vi "Day 2 task 1.vi"() -> ()   [LabVIEW 2022 SP3]
uses:
  <vilib>/regexp/Match Regular Expression.xnode
panel:
  out "sum":i32
  out "Array":i32[](array[numeric])
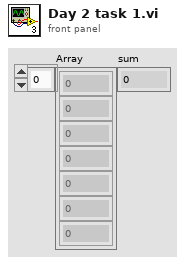
[diagram p1: front panel]
types:
  T1 = cluster{"Mine":string, "Theirs":string, "Score":i32}[]
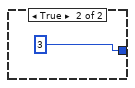
[diagram p2: hidden frame]
diagram:
  (unwired) "A Y\nB X\nC Z"
  w9 = TRUE ("replace all? (F)")
  n1 = Search and Replace String(replace all?=w9, input string="C Y\nC Y\nB Y\nA Z\nB Z\nA X\nA Y\nA Y\nA X\nA Y\nB Y\nA Y\nB Y\nB Y\nB Z\nB Z\nB Z\nB Z\nA Y\nB Z\nA Y\nB X\nB Y\nB X\nA X\nA X\nB Z\nA X\nA X\nB Z\nB Z\nB Y\nB Z\nB Z\nB Z\nB Y\nA X\nA X\nB Z\nA X\nB X\nB X\nC Y\nB Z\nC X\nA X\nA Y\nB Y\nA Y\nB X\nA X\nB Y\nB Z\nB Z\nB Y\nB Z\nC Z\nB X\nB X\nB Z\nB Z\nB Z\nB Z\nA Y\nB X\nA X\nC X\nB Y\nB Z\nA Y\nB Z\nB Z\nB Y\nB Y\nB Z\nB Y\nB Z\nA X\nB X\nB X\nA X\nA X\nB Z\nB Z\nB Z\nB Z\nB Y\nB X\nB Z\nA X\nA Y\nB Z\nA Y\nB Z\nB Y\nB Z\nA X\nB Y\nA Y\nB Z\nA Z\nA Y\nA Y\nC Y\nB Z\nB X\nA Z\nB Z\nA X\nB Z\nA Z\nB Z\nA X\nB Y\nA X\nB Y\nB Z\nB X\nB X\nB Z\nB Z\nB Z\nA X\nB Z\nA X\nB X\nB Z\nA X\nC Z\nB Z\nB Z\nB Y\nB Y\nB Y\nB Z\nB Z\nA Y\nB Z\nB Z\nC Y\nC Z\nA X\nB Z\nB X\nB Z\nB Z\nB Y\nA X\nB Z\nB Y\nA Z\nB Z\nA X\nA X\nB Y\nA Y\nB Z\nB Z\nB X\nB Y\nA X\nA Y\nB X\nC Z\nA Y\nB Z\nB Z\nB Z\nA Z\nC Y\nB Y\nB Y\nB Z\nC Y\nB Y\nB X\nB X\nB Z\nC Z\nA X\nB Z\nB Z\nB Z\nB Z\nB X\nB X\nA X\nA Z\nA Z\nA X\nC Y\nB X\nA X\nA Y\nA X\nB X\nA Y\nB Z\nB Z\nA Y\nA X\nB Y\nB Z\nB Z\nA X\nA Z\nB Z\nB X\nA X\nB Z\nB Y\nA Y\nA Z\nB X\nA Y\nB Z\nA Z\nB Z\nA Y\nB Z\nB X\nB Y\nA Y\nB Z\nB Z\nA X\nA X\nB Y\nB Z\nA X\nB Z\nB Z\nB Z\nB Z\nB Z\nA Z\nB Z\nB Z\nB X\nA Y\nC X\nB Z\nB Y\nB Y\nB Z\nB Z\nB Z\nB Y\nB X\nB Y\nC X\nB Z\nA Z\nA Y\nC X\nA X\nB X\nA X\nB X\nA Y\nB Z\nA Y\nA Y\nB Z\nB X\nB Z\nA Y\nB Z\nB X\nC Z\nC X\nC Z\nB Y\nB X\nB Z\nB Z\nB Y\nB Z\nB Y\nB Z\nA X\nB X\nB Z\nA X\nB Z\nB Y\nB Z\nA X\nB Y\nC Y\nA Z\nB Z\nC Z\nA Y\nB Z\nA Y\nA Z\nB Y\nA X\nA X\nB Z\nB Z\nB Z\nA Y\nB Z\nA Z\nB Z\nA Y\nA Z\nB Y\nC Z\nB Z\nA Z\nB X\nB Z\nB Y\nB Z\nA Z\nA Z\nB Z\nB X\nC Z\nB X\nB Z\nB Y\nA X\nB Z\nA X\nB X\nB Z\nB Z\nA X\nB X\nC X\nC X\nB X\nB Y\nB Z\nB X\nB Y\nB Y\nB Z\nA Z\nB Z\nC X\nA Y\nC X\nB Z\nA Y\nB Z\nB Y\nB Z\nB X\nA X\nB X\nB Z\nA Y\nA Y\nB Z\nB Z\nB Z\nA Y\nB Z\nB X\nC X\nB Z\nB Z\nC Y\nB Z\nC Y\nB Z\nC Y\nC X\nB Z\nC Y\nA Y\nA Y\nC Z\nB Z\nB X\nB Z\nB X\nC Z\nB Z\nA Z\nB Z\nC Y\nB Z\nA X\nA Y\nB Y\nB Y\nB Z\nA Y\nB X\nB Z\nB Z\nA Z\nB X\nA Y\nA Y\nB Z\nB Z\nB Z\nC X\nA Z\nB X\nC Z\nB Y\nB Z\nB X\nA Y\nB Z\nA X\nB X\nB Y\nA Y\nB Z\nB Z\nB Y\nA Z\nB Z\nA X\nB Y\nA Y\nA X\nA Y\nA X\nA X\nB X\nB Y\nB X\nB Y\nB Z\nB Y\nB X\nA X\nB Z\nA Z\nA X\nB Z\nB Y\nA X\nB Y\nA X\nB X\nC Y\nB X\nB X\nB X\nC Y\nB X\nB Y\nB Y\nB Y\nB Y\nB X\nA Y\nC Y\nB Z\nB Z\nB X\nB Z\nC Y\nB Y\nB Z\nB Z\nB Y\nB Z\nA X\nB X\nB Y\nA X\nC Y\nB Z\nA Y\nB Z\nB Z\nB Z\nA X\nB Y\nB Z\nB Y\nB Z\nA X\nB Z\nA X\nB Y\nB Y\nB X\nB X\nA Y\nB Z\nC Y\nA X\nA X\nB X\nB Z\nB X\nB X\nB Z\nB Z\nA X\nB X\nB Z\nA Z\nB Y\nA X\nB Z\nC Y\nB Z\nB X\nB Z\nB Z\nA Y\nA Y\nB Z\nB X\nB Y\nB Z\nA Y\nA Y\nB X\nB X\nC X\nB Z\nC Z\nB X\nA Y\nB Z\nA Z\nB Y\nA Y\nB Z\nB X\nB X\nA Y\nB Z\nB Y\nA X\nB Y\nB Y\nB Y\nB X\nB Y\nB Z\nB Y\nB Y\nA X\nC Z\nB Z\nB Z\nA Z\nB Z\nB Z\nA X\nB X\nA Y\nA X\nB X\nC X\nB X\nB Z\nB Y\nA Z\nA Y\nB Y\nB Z\nB X\nB X\nB Z\nB Z\nB Y\nA X\nB Z\nA Y\nA X\nB Y\nB Z\nB Z\nB X\nA X\nA Y\nC X\nA Y\nB Z\nB Y\nB Z\nB Z\nC Z\nB Z\nB X\nA X\nC Y\nB X\nB Z\nA Z\nA X\nA Y\nB Z\nB Z\nA Y\nA Y\nB X\nA Y\nA Y\nB Z\nA Y\nB Y\nB Z\nA Y\nA Z\nB X\nB X\nB Y\nB Z\nB Z\nA X\nB X\nC X\nB Y\nA Y\nA X\nA X\nA X\nB Y\nA X\nA Z\nA Y\nB X\nA Y\nB Z\nC X\nB X\nB X\nB Z\nB X\nB X\nB Z\nA X\nB Z\nB X\nB Z\nA Y\nB Y\nB Z\nB Y\nB Z\nB Z\nA X\nB Z\nA Y\nC Z\nA Y\nB Z\nA Y\nB X\nB Z\nB X\nC Y\nA X\nB Z\nB Y\nA X\nA X\nB X\nB Z\nA Z\nB Z\nB X\nB X\nB X\nB Z\nB Z\nB Y\nB X\nB X\nA X\nB Z\nB X\nA X\nA X\nA X\nB X\nB Z\nA Z\nB X\nB Y\nB Y\nB Z\nB Z\nC Z\nA Y\nA X\nB Y\nB X\nB Z\nB X\nA X\nB Z\nB Z\nB Y\nB Z\nB X\nB Z\nB Z\nB X\nB X\nA X\nA X\nB X\nB Z\nB Z\nC X\nC X\nB Z\nB Z\nB X\nB Z\nB Y\nB X\nA X\nB Y\nA Y\nA X\nB Z\nB Z\nC X\nB Y\nB Z\nB Z\nB X\nB Z\nB Z\nC Z\nB Z\nB Y\nB Z\nB X\nA X\nB X\nB Z\nB Z\nA Y\nB Z\nB Z\nB Z\nB Z\nA X\nB Z\nB Z\nB X\nB Y\nB Y\nB Z\nA X\nB Z\nB Y\nB X\nA X\nB X\nB Z\nB Z\nB Z\nB X\nB Z\nB Z\nB Z\nA Y\nB Z\nC X\nB Y\nB Y\nB Y\nA Y\nB Z\nB Z\nA X\nC Z\nB Z\nB Z\nB Z\nB X\nB Z\nA Z\nB Z\nB Z\nB Z\nA Z\nB Z\nC Y\nB X\nA X\nA Y\nB Z\nB Z\nA Z\nB Z\nB X\nA Z\nB Y\nB Z\nB X\nB Z\nB X\nB Y\nB Z\nA X\nB Z\nB Z\nA Y\nB X\nB X\nB X\nA Z\nC X\nA Z\nB Z\nB Z\nB Z\nB X\nA Y\nC X\nA Z\nA Y\nB X\nB Z\nB X\nB Z\nB Y\nA Y\nB X\nC X\nA Y\nC Z\nA X\nB Z\nB Z\nA Z\nB X\nB Y\nB Z\nA Y\nB Y\nA X\nA X\nC Y\nA Y\nB X\nA X\nB Y\nB X\nB Y\nA Y\nA X\nC Y\nB Y\nB Y\nB Z\nB Y\nB X\nB Z\nB Z\nB X\nA X\nB Z\nB Z\nB Z\nB X\nB Z\nB X\nB Z\nB Z\nB Y\nB Y\nB X\nA X\nB Z\nB Y\nA Y\nB Z\nB X\nB Z\nB Z\nA Z\nB Z\nA Y\nB Z\nA X\nB Z\nB Z\nA Y\nB Z\nA X\nB Z\nA Y\nA Y\nA Z\nB X\nB Z\nB Y\nA Z\nC Z\nB Z\nA X\nA X\nB X\nA Z\nB X\nB X\nB Z\nC X\nB Z\nB Z\nB Z\nB Z\nB X\nA Z\nA Y\nB Z\nB Y\nC Z\nB Y\nB Z\nA Y\nB X\nB X\nB Z\nA X\nA Y\nB Z\nB X\nB Y\nA Y\nC Y\nC Y\nB Z\nA Y\nB Y\nA Y\nB Z\nB Z\nA X\nB X\nA X\nB X\nA Y\nA X\nB Z\nA X\nB Z\nB X\nB Z\nB X\nB X\nA X\nA Y\nB Z\nB X\nB X\nA X\nA Y\nA X\nB Y\nB Z\nB Z\nB Z\nB Z\nB Z\nB X\nB Y\nA Y\nB X\nB Z\nA Y\nB X\nA X\nB Z\nC X\nB Y\nA Y\nA X\nA X\nB X\nB X\nB Z\nB Z\nB Z\nB X\nB Y\nB X\nB Z\nB X\nB Y\nB X\nB Z\nB X\nB Y\nB X\nB Z\nB Z\nB Z\nA X\nC X\nC Y\nA Y\nB X\nB X\nA Y\nB Z\nB X\nB Z\nB X\nB X\nC X\nB Z\nB Z\nB Y\nA Z\nA Z\nC X\nB X\nC Y\nB Z\nC X\nB Z\nA Y\nC Z\nB X\nB Y\nA Y\nB Y\nB X\nB Z\nA Y\nA Z\nC X\nB Z\nA X\nB X\nB Z\nC Z\nA Y\nB Z\nB Z\nA X\nA X\nB Z\nB Y\nC Z\nB Z\nB X\nB Z\nA X\nA X\nB Y\nA X\nB X\nA Y\nB Z\nA Y\nB Z\nA Y\nB Z\nA X\nB Y\nB Z\nB Z\nB Z\nA X\nA X\nB X\nB Z\nA X\nB Z\nA X\nA X\nB Z\nB Z\nB Z\nB X\nB Y\nB Z\nB Z\nB X\nB Z\nB Y\nB Z\nC Y\nB X\nC Z\nB Z\nB Z\nA Y\nB Z\nB X\nA Y\nB Z\nB X\nB Z\nB Z\nB Y\nB Z\nA Z\nA Y\nB Z\nB Z\nB Y\nA Y\nB Z\nA X\nB X\nA Z\nA X\nB X\nB Z\nB X\nB Z\nB Z\nB Y\nB Y\nB Z\nB Y\nB Z\nB Z\nA X\nB X\nB Y\nB Y\nC Z\nA X\nB Y\nA Y\nB Z\nB Z\nB Z\nC X\nB X\nA Z\nB Y\nA X\nC X\nB Z\nB Z\nB Z\nB Y\nA Y\nA Y\nB Y\nB Z\nB Z\nB Z\nC X\nA X\nB Z\nA Y\nB X\nB Z\nB Z\nB Z\nB Z\nB X\nB Y\nB Z\nB Z\nA Y\nC X\nA X\nB Z\nB Z\nA Y\nA Y\nB Z\nA Y\nB Y\nA X\nB Z\nB Z\nA Y\nB Z\nB Z\nA X\nA X\nB X\nB Z\nB Z\nA X\nB Z\nB Z\nC Y\nB Z\nA X\nB Z\nA X\nB Z\nA X\nB X\nA X\nA Y\nB Z\nB X\nA X\nB Z\nA X\nA Z\nB Z\nB Z\nB Z\nA Y\nB X\nA X\nB Y\nA Y\nB Z\nB Z\nB X\nB Z\nB X\nB X\nA X\nB Z\nA Y\nA X\nB X\nA Z\nB X\nB Y\nB Z\nB X\nB X\nB Z\nC X\nA X\nB Z\nB Y\nC Z\nB Z\nA Z\nA Z\nA X\nA Y\nB Z\nB Z\nB X\nA Z\nB Z\nB Z\nB X\nB Y\nB X\nB Z\nB X\nB Z\nA Y\nA X\nB Z\nB X\nB Y\nB Z\nB Z\nB Z\nB Z\nC X\nC X\nB Z\nB X\nB Z\nB Z\nB Z\nB X\nB Z\nB Z\nB Z\nB X\nB Z\nB Z\nB Z\nC Y\nB Z\nB Y\nB Z\nA Z\nA Y\nB Z\nA Y\nC X\nA X\nB X\nA Y\nB Z\nA Y\nB Z\nB Y\nB Z\nB Z\nC Y\nB Y\nB Z\nB Z\nB X\nB Y\nB Z\nB Y\nB Z\nB X\nB Y\nB Z\nB Z\nB Z\nB Y\nB Y\nB Z\nB Z\nC X\nB Z\nA Y\nB Z\nB Z\nB Y\nB Y\nB Z\nB Z\nA Y\nB Z\nA Z\nC X\nA Y\nA Y\nA X\nB Z\nA X\nC Y\nA Z\nC Y\nC X\nB Z\nA X\nA Y\nB Z\nB Z\nB Z\nB Z\nB Y\nA Z\nA Y\nB Y\nA Y\nA Z\nB X\nB Z\nB Z\nA X\nC Y\nB Z\nB X\nC X\nA Z\nB Z\nB X\nB Y\nA X\nA X\nB Z\nC X\nB Z\nB Z\nB X\nB Z\nB Z\nB Z\nA X\nB Z\nB Y\nB Z\nB Z\nB Y\nB X\nA X\nB Z\nA X\nA X\nB Y\nB Z\nB X\nA Y\nC X\nB Y\nA X\nA X\nA X\nC Y\nB X\nC Z\nA X\nB Z\nA Z\nB Z\nA X\nA Y\nB Z\nA X\nB X\nA Y\nA X\nA Y\nB X\nB Y\nB Z\nB Y\nC X\nC Y\nB Z\nB Y\nB Z\nA X\nC Z\nB Z\nA X\nB X\nA X\nB X\nB Z\nB X\nB Z\nB Z\nB Z\nA X\nA X\nB Z\nB X\nB Z\nB Z\nB Z\nA X\nB Z\nB X\nA X\nC Z\nA Y\nB Z\nA Y\nB Z\nB Z\nB Z\nC Z\nB Z\nB Z\nA X\nB X\nA X\nB X\nA X\nB Z\nB Z\nB X\nB Z\nA X\nA Y\nA Y\nA Y\nB Z\nB Z\nB Z\nB Z\nA X\nB Z\nB Z\nB Y\nB Z\nA Z\nB Z\nA Y\nB Y\nB Y\nC Y\nB X\nB Z\nB Y\nB Z\nB Y\nB Z\nB Z\nA Y\nB X\nA Z\nB Z\nA X\nB Y\nA X\nB Z\nB Y\nA X\nB X\nB Z\nB Z\nB Z\nA Y\nA Y\nA X\nA Y\nA Y\nB X\nB Z\nB Y\nB Y\nB X\nB Y\nB X\nB X\nB X\nB Z\nB Z\nB Z\nA Y\nA Z\nB Y\nC X\nB X\nB Z\nC Y\nB Z\nC Y\nB Z\nB Z\nB Z\nB X\nA X\nB Z\nB Z\nA X\nB Z\nB Z\nB Z\nB Z\nB Z\nB Z\nB X\nA X\nA Y\nB Y\nB Z\nB Y\nB X\nA Z\nA X\nB X\nB Y\nB Z\nB Z\nB Z\nB X\nC X\nB X\nA Z\nA X\nA Y\nB Z\nB Z\nA X\nB Z\nA Y\nB X\nB Z\nB Y\nB Y\nA X\nB X\nB Z\nB Z\nB Z\nB Z\nB Y\nA Z\nA Y\nB X\nA X\nB Y\nB Z\nC Y\nB Z\nB Z\nB X\nA Z\nA Y\nB Y\nB Z\nA Y\nB Y\nA Y\nA X\nA Y\nB Y\nC X\nC Z\nB X\nA Z\nA X\nB Y\nB X\nA X\nB Z\nA Y\nA Z\nB Z\nB Z\nB Z\nA X\nB Z\nB Y\nB Z\nA X\nA Y\nB Z\nB X\nC X\nB Z\nA Y\nB Z\nB Z\nB X\nB Z\nB Z\nA Y\nA X\nB Z\nC Y\nA Y\nB Y\nB Z\nA X\nB Z\nB Z\nB Z\nB Z\nC X\nB Y\nB Z\nB X\nB Z\nB Z\nB Z\nB Z\nB Z\nB Y\nA X\nB Y\nA Y\nA X\nA X\nB Z\nB Z\nB Z\nC X\nB X\nB Z\nA X\nA X\nB Y\nA X\nB Z\nB Z\nB X\nB Y\nB Y\nB Y\nA Y\nA Y\nA X\nA X\nB Z\nB Y\nB Y\nB X\nB Y\nB Z\nA Z\nB Z\nA Z\nB X\nB Y\nC Y\nB X\nB X\nA X\nA X\nA X\nA X\nB Z\nB Z\nA Z\nB X\nB X\nB X\nB X\nB X\nB Z\nB Z\nB Z\nB Z\nB Z\nB Y\nB Z\nB Z\nA Y\nA Z\nC Y\nB Y\nA X\nB Z\nB X\nA Y\nB Y\nA Y\nC Z\nA X\nA Y\nB X\nB X\nC Z\nB Y\nA Y\nA Y\nA X\nB X\nA X\nB X\nA Y\nB Z\nB Z\nA Z\nB X\nB Z\nB Z\nB Y\nA Y\nB Z\nB Y\nB Z\nB Z\nB Z\nC X\nB Y\nA Y\nB Z\nA Y\nA Y\nA X\nB X\nB Y\nC Y\nC X\nB Z\nB Z\nB Z\nA Y\nA Z\nB Y\nB X\nB X\nB Y\nB Z\nB Z\nA Y\nB Y\nB Z\nB Z\nB Z\nA X\nC Y\nB Z\nA Z\nC Z\nB X\nB Y\nB Z\nA Z\nA X\nB X\nA X\nC X\nB Z\nA X\nB Y\nC Y\nB Y\nB Z\nB X\nA Y\nB Z\nB Z\nB Z\nA X\nB Z\nB Z\nB Z\nB Z\nA X\nB Z\nB X\nB X\nB Z\nC X\nA Y\nB Z\nB X\nB Z\nB Y\nB Z\nB Y\nC Y\nA X\nB Y\nB Z\nB Z\nB X\nB Z\nA X\nB Z\nA X\nB Y\nB Z\nA X\nB Z\nB X\nA Z\nB Z\nC X\nB Z\nB Y\nB Y\nB Y\nB Z\nB X\nB X\nA X\nA X\nB Z\nB Z\nA X\nA X\nA Z\nA Y\nC Z\nB Z\nB Y\nC X\nB X\nB Y\nB Y\nA Y\nB Z\nB Z\nB Y\nC Y\nB Z\nA Y\nB Z\nB Z\nB Z\nB Z\nA Y\nB Z\nB Z\nB Z\nA X\nB X\nA Y\nB Y\nB Z\nB Z\nB Z\nA Y\nB Z\nB Z\nB Z\nB Y\nB Y\nB X\nB X\nB Y\nC Z\nB X\nB Y\nC Y\nA Y\nB Z\nA Z\nB Z\nA Y\nB X\nB Z\nB X\nC Z\nA Y\nB X\nB Z\nA X\nA X\nB Z\nB Z\nB Y\nB Z\nC Y\nC X\nB Z\nB Z\nA X\nB X\nA Y\nB Y\nB Y\nC Z\nA X\nB X\nB Z\nA Y\nB Z\nC X\nB Z\nA Z\nC X\nA Y\nA Z\nB Z\nA Y\nA X\nB Z\nB Y\nB Z\nB X\nB Z\nA X\nB Z\nA Z\nB Z\nB Z\nB Y\nA X\nB Z\nB X\nB Y\nB Y\nA Y\nA X\nC Z\nB Y\nC Z\nA X\nB X\nB Z\nB X\nC X\nB Z\nB Z\nA X\nA Y\nA Z\nA Z\nB Z\nB Z\nA X\nB Z\nB Y\nA X\nA Y\nB Z\nB X\nA Y\nB Z\nB Y\nB X\nB Z\nA Z\nB Y\nA Y\nA X\nB Z\nB Z\nB Z\nB Z\nA X\nB Y\nB Z\nB Z\nB Z\nA Z\nB Y\nA X\nC Y\nB Z\nB Z\nB Y\nB X\nB Z\nA Y\nA X\nB Z\nB Y\nB Z\nA Y\nC X\nB Y\nB Z\nB Z\nA Y\nB X\nB Z\nB Z\nA X\nB X\nB Z\nA Z\nB Y\nB Z\nB Z\nB Z\nB Z\nB Z\nA Z\nB X\nA Y\nC Y\nB Z\nA Y\nB Z\nB Z\nA Y\nB Z\nB Z\nA Y\nA Y\nB X\nB Y\nA X\nB Z\nA Y\nB Z\nA Z\nB Z\nB X\nB Z\nB Z\nB Y\nB Y\nB Z\nA X\nB Y\nB Z\nB Z\nB Z\nB Y\nA Y\nB Z\nB Y\nB Z\nB Z\nB X\nA X\nB Y\nA X\nA X\nB Z\nA X\nB Z\nC X\nB Y\nB Z\nB Z\nB Y\nA X\nB Z\nB Z\nB Y\nB X\nB Z\nB X\nB Z\nC Y\nB Y\nB Z\nB Z\nA Z\nB Z\nB Z\nA Y\nB Z\nB Y\nA X\nB Z\nB Z\nB Z\nB X\nB Z\nB Y\nB Z\nB X\nC Z\nB Y\nB Z\nB Z\nB Y\nA X\nA X\nB Y\nA Y\nB Z\nB X\nB Y\nB Z\nB Y\nB Z\nA X\nC X\nB Z\nA Z\nC Y\nA X\nB Y\nB Y\nA X\nA X\nB Y\nB Z\nC Y\nB Z\nB Y\nA X\nB Y\nB Y\nB Z\nB X\nB Z\nC X\nC Y\nB X\nA Y\nB Z\nB Z\nB Z\nA X\nB Z\nB Z\nB X\nB X\nB X\nB X\nB Y\nA Y\nB Z\nB Z\nB Z\nA Z\nB X\nB X\nB X\nB X\nB Z\nA Y\nB Y\nB Z\nA X\nA X\nA X\nB Y\nB Z\nB X\nB Z\nA Z\nB Z\nB Z\nA Y\nC Z\nA X\nB Z\nC X\nB Z\nB Z\nB Z\nB Y\nB Y\nB Z\nC X\nB Z\nA Y\nB X\nC X\nA Y\nC X\nB Z\nB X\nA Z\nB Z\nC Y\nB Y\nB X\nB Z\nB Y\nA Y\nB X\nA Z\nB Z\nB Z\nC Z\nB Z\nB Y\nB Z\nA Y\nC Y\nB Z\nB X\nA Y\nB Z\nB Z\nB Y\nB Y\nB Z\nA X\nA Y\nA X\nA Z\nB Z\nB Z\nB Y\nA Y\nB Y\nB Z\nB Y\nA Y\nB X\nA X\nB Y\nB Y\nB X\nB Z\nB Y\nC X\nB Z\nB Z\nB Z\nA X\nB Z\nB X\nA Y\nA Y\nB Z\nA Y\nA Y\nA Y\nB Y\nB Z\nA X\nC X\nB Y\nA X\nC X\nB Z\nB Y\nA Y\nB X\nB Z\nB Y\nB Y\nB Z\nB Z\nA Y\nB X\nB X\nA X\nB Z\nB X\nB Z\nB Z\nC Z\nC Y\nA X\nB X\nC X\nB X\nA Z\nA X\nB Y\nC X\nB Y\nA X\nA X\nA X\nB X\nB Z\nB X\nB Y\nB Z\nB Z\nB Z\nB Z\nA X\nA X\nB X\nB Z\nA Z\nA X\nB Z\nC Y\nB Z\nA X\nB Z\nA Z\nB Z\nB Z\nA Y\nB Y\nB Z\nB X\nB Z\nB Z\nC Y\nB Z\nB X\nA X\nB Y\nB Z\nA Y\nA X\nB Z\nB Y\nB Z\nB X\nA Y\nC Z\nB X\nB Z\nA X\nB X\nB Z\nB Z\nA X\nB Y\nB X\nB Z\nB Z\nB Y\nB X\nB X\nC X\nB Z\nC X\nB Z\nC Y\nA Y\nC X\nB X\nB Y\nB Z\nB Y\nB Z\nA X\nB Z\nB Z\nB Y\nB Y\nA X\nA X\nA Y\nB Z\nB Z\nA Y\nB Z\nA X\nB Z\nB X\nB X\nB X\nA Y\nB Z\nB Z\nA Y\nB Z\nA Z\nB Y\nB X\nA Z\nA Z\nB Z\nA Y\nB Z\nB Y\nB Y\nB X\nA Y\nB X\nB Z\nB Z\nB Y\nB X\nB Z\nB Z\nB Z\nB Z\nA X\nB X\nB X\nB Z\nA X\nB X\nB Z\nB Z\nB Y\nA Y\nB Z\nB Y\nB Y\nA X\nB X\nB Y\nC X\nC X\nB Y\nA Y\nA Z\nB X\nB Z\nB Z\nB Z\nB Z\nA X\nA Y\nA Y\nB Y\nC X\nB Z\nA Y\nB X\nC Z\nB X\nB Y\nA Y\nB X\nB Y\nB Z\nB Y\nB X\nB Y\nA Z\nB Z\nA X\nB X\nB X\nB Z\nB Y\nB Y\nB Y\nA X\nB X\nB Y\nB Z\nA Y\nA X\nB X\nB Z\nB Z\nC X\nA Z\nB Z\nA X\nA Y\nC X\nB Z\nB Z\nA X\nB X\nA Y\nA Y\nB Z\nB Z\nB X\nA Z\nB Z\nB Y\nA Y\nB Z\nB Y\nA Y\nB Y\nB Z\nA X\nB Y\nA X\nA Y\nA X\nA X\nB Y\nA Z\nB Z\nA Y\nB Z\nA Z\nA Y\nB Z\nB Y\nB Z\nB X", search string="A", replace string="R" ("replace string (\"\")"), error in=errorcluster {"status"=FALSE, "code"=0, "source"=""}) -> (result string=w27:string, error out=w21:errorcluster)  [unwired: 3 in, 2 out]
  n2 = Search and Replace String(replace all?=w9, input string=w27, search string="B", replace string="P" ("replace string (\"\")"), error in=w21) -> (result string=w23:string, error out=w20:errorcluster)  [unwired: 3 in, 2 out]
  n3 = Search and Replace String(replace all?=w9, input string=w23, search string="C", replace string="S" ("replace string (\"\")"), error in=w20) -> (result string=w7:string, error out=w8:errorcluster)  [unwired: 3 in, 2 out]
  n4 = Search and Replace String(replace all?=w9, input string=w7, search string="X", replace string="R" ("replace string (\"\")"), error in=w8) -> (result string=w12:string, error out=w18:errorcluster)  [unwired: 3 in, 2 out]
  n5 = Search and Replace String(replace all?=w9, input string=w12, search string="Y", replace string="P" ("replace string (\"\")"), error in=w18) -> (result string=w16:string, error out=w19:errorcluster)  [unwired: 3 in, 2 out]
  n6 = Search and Replace String(replace all?=w9, input string=w16, search string="Z", replace string="S" ("replace string (\"\")"), error in=w19) -> (result string=w6:string, error out=w5:errorcluster)  [unwired: 3 in, 2 out]
  n7 = Spreadsheet String To Array(delimiter (Tab)="\n", format string="%s", spreadsheet string=w6, array type (2D Dbl)=string[] []) -> (array=w31:string[])
  n8 = for {
    tunnel: w31 -> [w46] mode=indexing
    tunnel: w5 -> [w45]
    tunnel: cluster{"Mine":string, "Score":i32}[] [{"Mine"="R", "Score"=1}, {"Mine"="P", "Score"=2}, {"Mine"="S", "Score"=3}] -> [w40]
    tunnel: T1 [{"Mine"="R", "Theirs"="P", "Score"=0}, {"Mine"="R", "Theirs"="S", "Score"=6}, {"Mine"="P", "Theirs"="R", "Score"=6}, {"Mine"="P", "Theirs"="S", "Score"=0}, {"Mine"="S", "Theirs"="R", "Score"=0}, {"Mine"="S", "Theirs"="P", "Score"=6}] -> [w37]
    tunnel: [w39] -> w2 mode=indexing
    n9 = xnode "Match Regular Expression"("input string"=w46, "regular expression"="\\s", "error in"=w45) -> ("before match"=w41:string, "after match"=w36:string)  [unwired: 3 in, 3 out]
    n10 = Equal?(x=w41, y=w36) -> (x = y?=w43:bool)
    n11 = case shown="False" w43 {
      tunnel: [w52 3 ("x")] -> w42
      tunnel: w41 -> [w53 _]
      tunnel: w37 -> [w55 _]
      tunnel: w36 -> [w54 _]
      frame False {
        n12 = for {
          tunnel: w55 -> [w64] mode=indexing
          tunnel: w54 -> [w62]
          tunnel: w53 -> [w61]
          tunnel: [w56] -> w52
          stop <- w57 stop-if-true
          n13 = Unbundle(w64) -> ("Mine"=w63:string, "Theirs"=w60:string, "Score"=w56:i32)
          n14 = Equal?(x=w61, y=w60) -> (x = y?=w58:bool)
          n15 = Equal?(x=w62, y=w63) -> (x = y?=w59:bool)
          n16 = And(x=w58, y=w59) -> (x .and. y?=w57:bool)
        }
      }
      frame True {
      }
    }
    n17 = for {
      tunnel: w36 -> [w50]
      tunnel: w40 -> [w51] mode=indexing
      tunnel: [w47] -> w38
      stop <- w48 stop-if-true
      n18 = Unbundle(w51) -> ("Mine"=w49:string, "Score"=w47:i32)
      n19 = Equal?(x=w50, y=w49) -> (x = y?=w48:bool)
    }
    n20 = Add(x=w42, y=w38) -> (x+y=w39:i32)
  }
  "Array" <- w2
  n21 = Add Array Elements(numeric array=w2) -> (sum=→"sum":i32)
